vi "ResettableTimer.vi"(11 "Restart timer?":bool) -> (3 "Time since last reset":dbl)   [LabVIEW 2013]
doc: "This VI times how long it's been since the boolean was last triggered. After being triggered, the timer rezeros and then outputs the time since that triggering.\n\nEric Schneider, Jan. 2014"
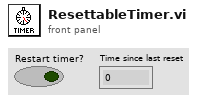
[diagram p1: front panel]
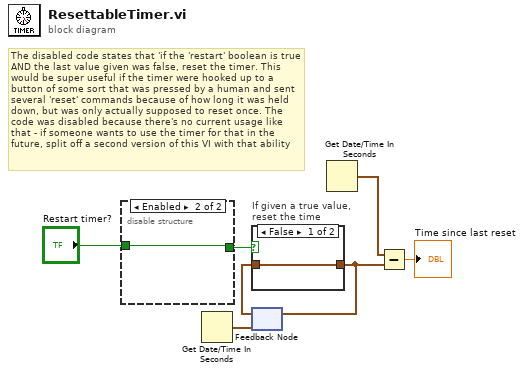
[diagram p0: block diagram]
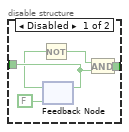
[diagram p2: hidden frame]
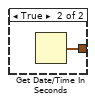
[diagram p3: hidden frame]
diagram:
  # "The disabled code states that 'if the 'restart' boolean is true AND the last value given was false, reset the timer. This would be super useful if the timer were hooked up to a button of some sort that was pressed by a human and sent several 'reset' commands because of how long it was held down, but was only actually supposed to reset once. The code was disabled because there's no current usage like that - if someone wants to use the timer for that in the future, split off a second version of this VI with that ability"
  n1 = disable-structure shown="Enabled" {
    disable-tunnel: "Restart timer?" -> [w12 w13]
    disable-tunnel: [w8 w13] -> w4
    frame Disabled {
      n2 = feedback #1(FALSE ("InIrons?")) -> (w9:bool)
      n3 = Not(x=w9) -> (.not. x?=w11:bool)
      n4 = feedback-in #1(w12) -> ()
      n5 = And(x=w11, y=w12) -> (x .and. y?=w8:bool)
    }
    frame Enabled {
    }
  }
  n6 = Get Date/Time In Seconds() -> (seconds since 1Jan1904=w2:timestamp)
  n7 = feedback #2(w2) -> (w3:timestamp)
  n8 = case "If given a true value,\nreset the time" shown="False" w4 {
    tunnel: [w14 w15] -> w1
    tunnel: w3 -> [w14 _]
    frame False {
    }
    frame True {
      n9 = Get Date/Time In Seconds() -> (seconds since 1Jan1904=w15:timestamp)
    }
  }
  n10 = feedback-in #2(w1) -> ()
  n11 = Get Date/Time In Seconds() -> (seconds since 1Jan1904=w5:timestamp)
  n12 = Subtract(x=w5, y=w1) -> (x-y=→"Time since last reset":dbl)
